vi "sv_Convert Numeric to Array of Digits of Base X.vi"(5 "fixed width":i32=-1 min=-1 max=51 step=1, 7 "base":u8=16 min=2 max=16 step=1, 11 "numeric":u64) -> (3 "byte array":u8[](array[numeric]) format="%.0x")   [LabVIEW 2017]
doc: "Use this subVI to convert a numeric into a byte array. Each element corresponds to a digit of the input numeric in the specified base."
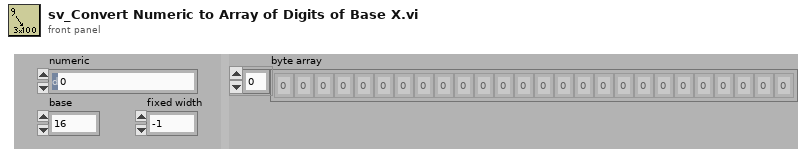
[diagram p1: front panel]
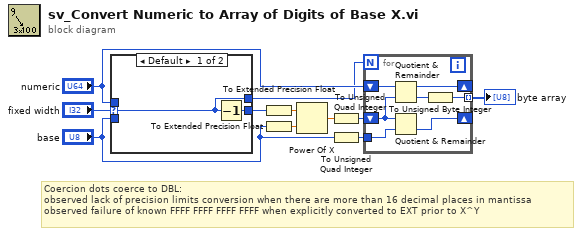
[diagram p0: block diagram]
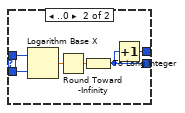
[diagram p2: hidden frame]
diagram:
  # "Coercion dots coerce to DBL:\nobserved lack of precision limits conversion when there are more than 16 decimal places in mantissa\nobserved failure of known FFFF FFFF FFFF FFFF when explicitly converted to EXT prior to X^Y"
  n1 = case shown="Default" "fixed width" {
    selector: "fixed width" -> [w13 _]
    tunnel: "numeric" -> [_ w19]
    tunnel: [w12 w15] -> w2
    tunnel: "base" -> [_ w16]
    tunnel: [w13 w14] -> w1
    frame Default {
      n2 = Decrement(x=w13) -> (x-1=w12:i32)
    }
    frame ..0 {
      n3 = Logarithm Base X(1:w16, 2:w19) -> (0:w18:dbl)
      n4 = Round Toward -Infinity(1:w18) -> (0:w17:dbl)
      n5 = To Long Integer(number=w17) -> (32bit integer=w15:i32)
      n6 = Increment(x=w15) -> (x+1=w14:i32)
    }
  }
  n7 = To Extended Precision Float(1:w2) -> (0:w5:ext)
  n8 = To Extended Precision Float(1:"base") -> (0:w4:ext)
  n9 = Power Of X(1:w4, 2:w5) -> (0:w7:ext)
  n10 = To Unsigned Quad Integer(1:w7) -> (0:w10:u64)
  n11 = To Unsigned Quad Integer(1:"base") -> (0:w8:u64)
  n12 = for {
    N: w1 -> [_]
    shift-right: [w25] -> _
    shift-left: "numeric" -> [w26]
    tunnel: w8 -> [w23]
    shift-right: [w24] -> _
    shift-left: w10 -> [w22]
    tunnel: [w20] -> w9 mode=indexing
    n13 = Quotient & Remainder(x=w26, y=w22) -> (x-y*floor(x/y)=w25:u64, floor(x/y)=w21:u64)
    n14 = Quotient & Remainder(x=w22, y=w23) -> (floor(x/y)=w24:u64)  [unwired: 1 out]
    n15 = To Unsigned Byte Integer(number=w21) -> (unsigned 8bit integer=w20:u8)
  }
  "byte array" <- w9
